vi "Loader Management Core.vi"(9 "Loader Name Override":string, 10 "Plugin Loader Path Override":path, 11 "CIFPluginManager in":refnum<class "CIFPluginManager.lvclass">) -> (0 "error out":errorcluster)   [LabVIEW 2021, in "CIFPluginManager.lvclass"]
uses:
  CIFPluginManager.lvclass
  CIFPluginManager.lvclass/CIFPluginManager.ctl
  typedef/Loader Load Command.ctl
  typedef/Loader Type.ctl
  <vilib>/CIF Foundation/CIF Core/CIFUtilities/CIFLogs/Logs/Write Error.vi
  <vilib>/CIF Foundation/CIF Core/CIFPluginManager/gRPC/CIF_Manager_Client_Wrapper/CIFManagerClientWrapper.lvlib
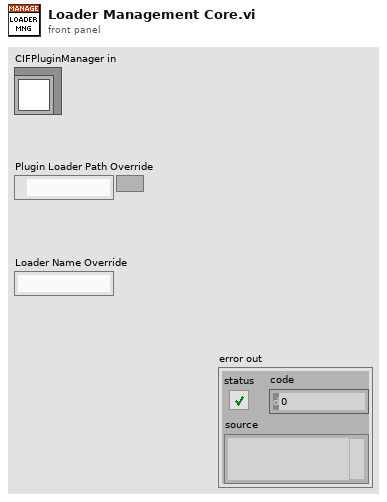
[diagram p1: front panel]
types:
  T1 = typedef "CIFPluginManager.lvclass/Loader Load Command.ctl" = cluster{"Loader Type":T2, "Loader Name":string}
  T2 = typedef "CIFPluginManager.lvclass/Loader Type.ctl" = enum16{"LabVIEW"}
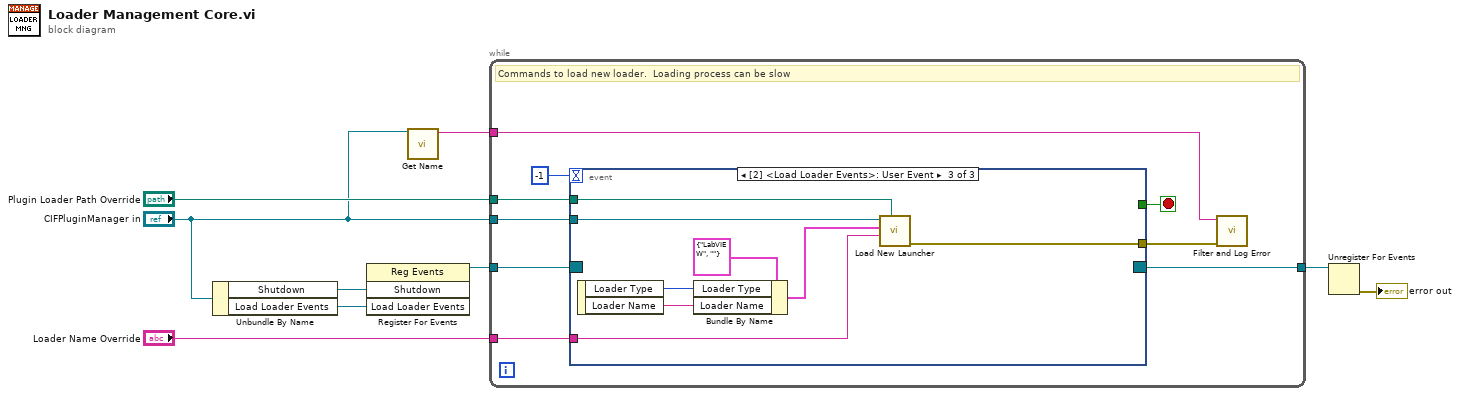
[diagram p0: block diagram]
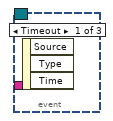
[diagram p2: hidden frame]
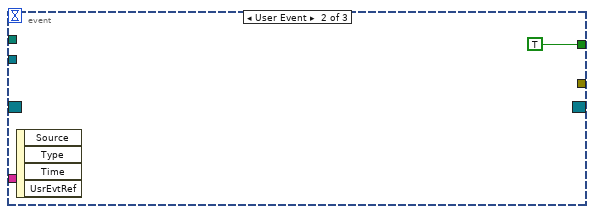
[diagram p3: hidden frame]
diagram:
  n1 = Unbundle By Name("CIFPluginManager in") -> ("Shutdown"=w6:refnum<user-event>, "Load Loader Events"=w7:refnum<user-event>)
  n2 = register-events(w6, w7) -> (reference out=w5:refnum<event-registration>)  [unwired: 2 in, 1 out]
  n3 = call "Get Name.vi"("CIFPluginManager in"="CIFPluginManager in") -> ("Name"=w1:string)  [unwired: 10 in]
  n4 = while {
    tunnel: w5 -> [w18]
    tunnel: [w14] -> w8
    tunnel: "Plugin Loader Path Override" -> [w12]
    tunnel: "Loader Name Override" -> [w11]
    tunnel: "CIFPluginManager in" -> [w17]
    tunnel: w1 -> [w10]
    stop <- w15 stop-if-true
    # "Commands to load new loader.  Loading process can be slow"
    n5 = event shown="[2] <Load Loader Events>: User Event" {
      selector: w18 -> [_ _ _]
      dyn-events: [_ _ _] -> w14
      timeout: -1 -> [_ _ _]
      tunnel: w17 -> [_ _ w27]
      tunnel: [_ TRUE _] -> w15
      tunnel: [_ _ w26] -> w13
      tunnel: w12 -> [_ _ w21]
      tunnel: w11 -> [_ _ w20]
      event Timeout {
        n6 = event-data() -> ()  [unwired: 1 in, 3 out]
      }
      event User Event {
        n7 = event-data() -> ()  [unwired: 1 in, 4 out]
      }
      event User Event {
        n8 = event-data() -> ("Loader Type"=w24:T2, "Loader Name"=w23:string)  [unwired: 1 in]
        n9 = Bundle By Name(cluster=T1 {"Loader Type"=enum."LabVIEW", "Loader Name"=""} ("Launcher Load Info"), "Loader Type"=w24, "Loader Name"=w23) -> (w22:T1)
        n10 = call "Load New Launcher.vi"("Plugin Loader Path Override"=w21, "Loader Name Override"=w20, "Loader Load Info"=w22, "CIFPluginManager in"=w27) -> ("error out"=w26:errorcluster)  [unwired: 7 in]
      }
    }
    n11 = call <vilib>:"Filter and Log Error.vi"("error In"=w13, "Name"=w10) -> ()  [unwired: 10 in]
  }
  n12 = Unregister For Events(event registration refnum=w8) -> (error out=→"error out":errorcluster)  [unwired: 1 in]
